vi "emballage affiche l'historique.vi"() -> ()   [LabVIEW 2020]
doc: "Affiche les pièces du même type que le produit scanné mais qui ont déjà été emballées (champ date d'emballage non vide)"
uses:
  Modules/FS/60_FS_Controles/60_FS_SetGet.ctl
  <vilib>/Utility/miscctls.llb/LVRowAndColumnUnsignedTypeDef.ctl
panel:
  in  "No Pièce":string caption="Entrez le No de la pièce que vous voulez chercher et cliquez sur Enter"
  in  "quitter":bool
  out "Pièces déjà emballées (Historique)":i32(listbox)
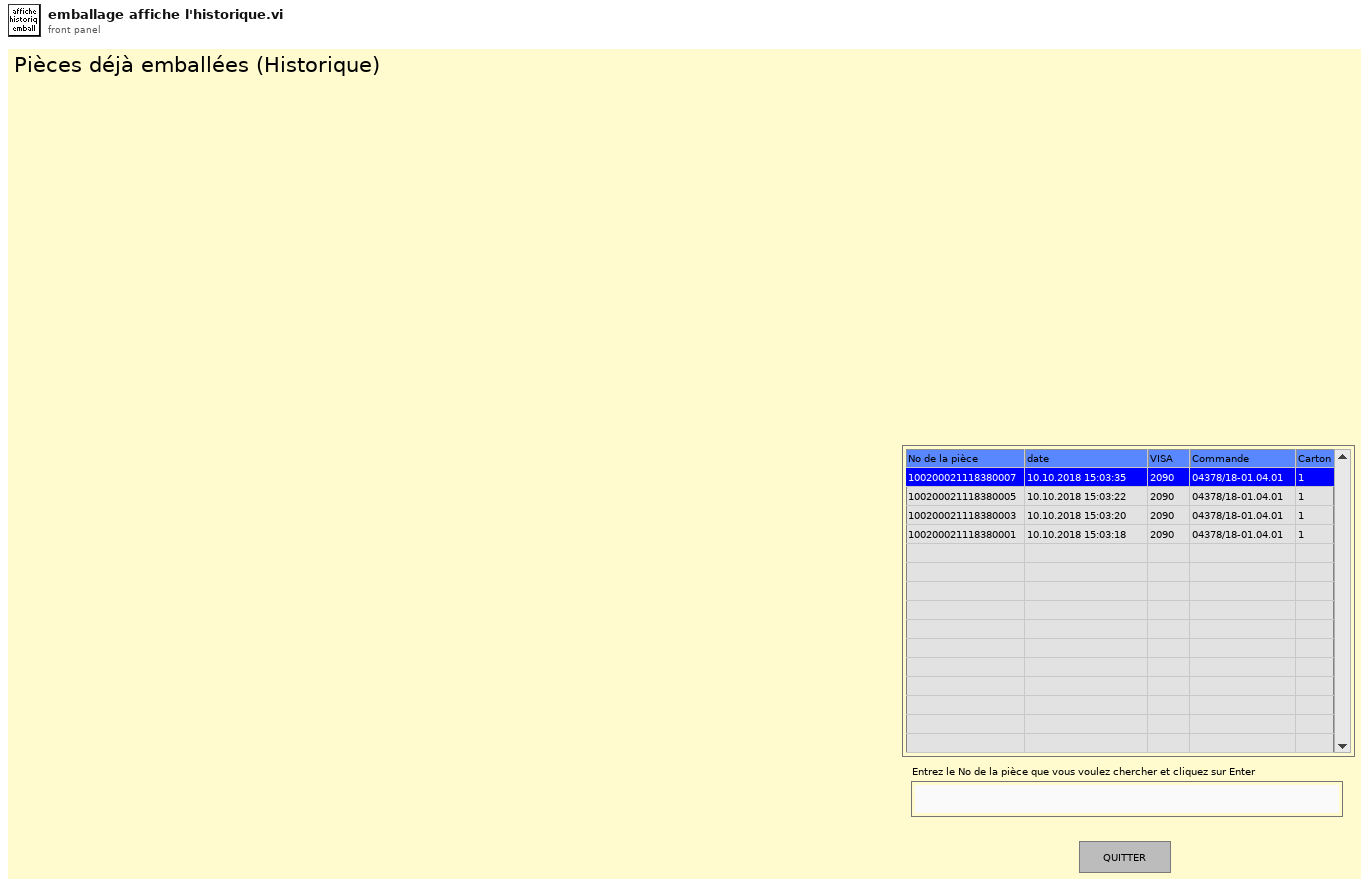
[diagram p1: front panel]
types:
  T1 = typedef "LVRowAndColumnUnsignedTypeDef.ctl" = cluster{"Row":u32, "Column":u32}
  T2 = typedef "60_FS_SetGet.ctl" = enum16{"set", "get"}
  T3 = typedef "Emballage_BDD_param_Produit.ctl" = cluster{"No_Valve_FAS":string, "suffixe":string, "designation":string, "indice_produit":string, "code_barre_fixe":string, "affiche_code_barre_client":string, "affiche_no_client":string, "Nb_vlve_par_carton":u16, "melange_des_lots_possible":string, "id_article":string, "Indice_Rev":string, "Famille":string, "date":string, "code_barre_fixe_Fin":string, "Longeur_No_Serie":string}
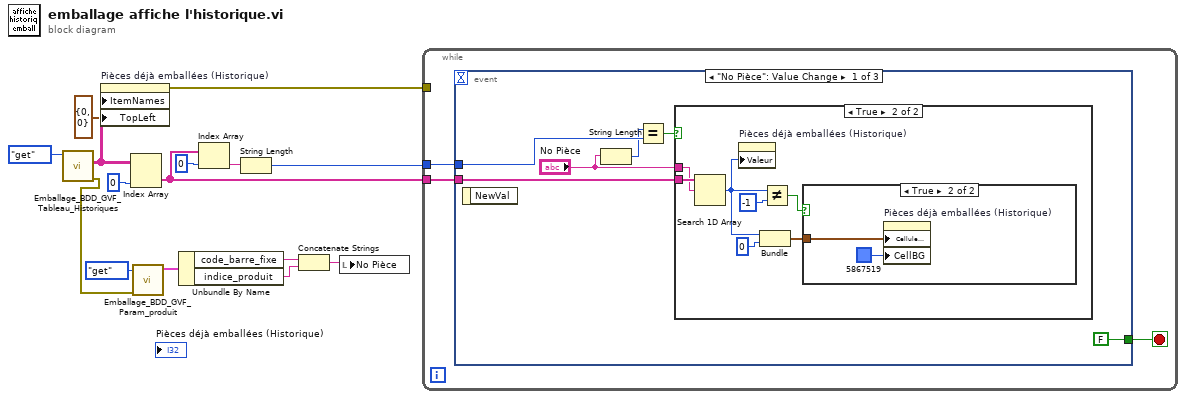
[diagram p0: block diagram]
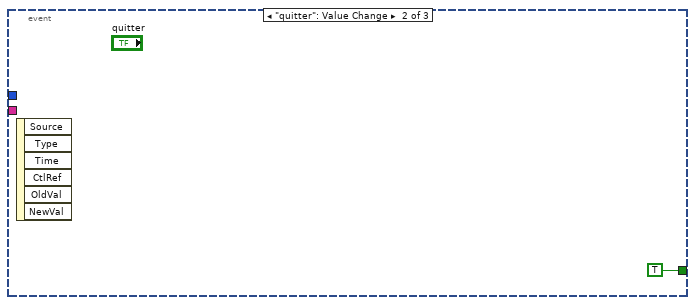
[diagram p4: hidden frame]
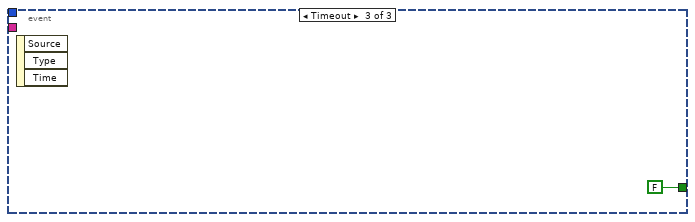
[diagram p5: hidden frame]
diagram:
  n1 = call "Emballage_BDD_GVF_Tableau_Historiques.vi"("SetGet"=60_FS_SetGet."get") -> ("Error out"=w1:errorcluster, "Tableau historique OUT"=w13:string[][])  [unwired: 9 in]
  n2 = property on="Pièces déjà emballées (Historique)" class="MCListbox (strict)"("ItemNames"=w13, "TopLeft"=T1 {"Row"=0, "Column"=0} ("Cellule visible en haut à gauche")) -> (error out=w15:errorcluster)  [unwired: 2 in, 1 out]
  n3 = Index Array(array=w13, index (col)=0 ("indice désactivé (col)")) -> (element=w11:string[])  [unwired: 1 in]
  n4 = call "Emballage_BDD_GVF_Param_produit.vi"("Error in"=w1, "Énum"=enum16{"set", "get"}."get") -> ("CLS_param_produit"=w3:T3)  [unwired: 6 in, 3 out]
  n5 = Unbundle By Name(w3) -> ("code_barre_fixe"=w4:string, "indice_produit"=w5:string)
  n6 = Index Array(array=w11, index=0 ("indice")) -> (element=w9:string)
  n7 = String Length(string=w9) -> (length=w8:i32)
  n8 = Concatenate Strings(w4, w5) -> (w2:string)
  n9 = local write "No Pièce"(w2) -> ()
  n10 = while {
    tunnel: w15 -> [_]
    tunnel: w11 -> [w18]
    tunnel: w8 -> [w17]
    stop <- w16 stop-if-true
    n11 = event shown="[0] \"No Pièce\": Value Change" {
      selector: _ -> [_ _ _]
      dyn-events: _ -> [_ _ _]
      timeout: _ -> [_ _ _]
      tunnel: w18 -> [w24 _ _]
      tunnel: w17 -> [w22 _ _]
      tunnel: [FALSE ("quitter") TRUE ("quitter") FALSE ("quitter")] -> w16
      event "No Pièce": Value Change {
        n12 = event-data() -> ()  [unwired: 1 in, 1 out]
        n13 = String Length(string="No Pièce") -> (length=w20:i32)
        n14 = Equal?(x=w20, y=w22) -> (x = y?=w23:bool)
        n15 = case shown="True" w23 {
          tunnel: w24 -> [_ w31]
          tunnel: "No Pièce" -> [_ w25]
          frame False {
          }
          frame True {
            n16 = Search 1D Array(1D array=w31, element=w25) -> (index of element=w27:i32)  [unwired: 1 in]
            n17 = property on="Pièces déjà emballées (Historique)" class="MCListbox (strict)"("Valeur"=w27) -> ()  [unwired: 2 in, 2 out]
            n18 = Bundle("index of element"=w27, 0) -> (w29:cluster{"index of element":i32, i32})  [unwired: 1 in]
            n19 = Not Equal?(x=w27, y=-1) -> (x != y?=w26:bool)
            n20 = case shown="True" w26 {
              tunnel: w29 -> [_ w33]
              frame False {
              }
              frame True {
                n21 = property on="Pièces déjà emballées (Historique)" class="MCListbox (strict)"("Cellule visible en haut à gauche"=w33, "CellBG"=u32 5867519) -> ()  [unwired: 2 in, 2 out]
              }
            }
          }
        }
      }
      event "quitter": Value Change {
        n22 = event-data() -> ()  [unwired: 1 in, 6 out]
      }
      event Timeout {
        n23 = event-data() -> ()  [unwired: 1 in, 3 out]
      }
    }
  }
